vi "log analysis_gps.vi"() -> ()   [LabVIEW 2019] (continued)
0.0929,0.0781,0.0970,0.1019,4.9840,0f000001,0*955fd833\n\t", "INSPVAXA,USB3,0,45.5,FINESTEERING,2107,283346.950,02000000,471d,15824;INS_ALIGNMENT_COMPLETE,INS_RTKFIXED,37.37118779202,126.72299929144,7.7854,22.3000,0.1003,-0.2796,-0.0183,-0.357856906,-0.723006737,278.633509270,0.4452,0.2974,0.5713,0.1136,0.0929,0.0781,0.0970,0.1019,4.9840,0f000001,0*7a9ec2a9\n\t", "INSPVAXA,USB3,0,50.5,FINESTEERING,2107,283347.450,02000000,471d,15824;INS_ALIGNMENT_COMPLETE,INS_RTKFIXED,37.37118807403,126.72299804089,7.7866,22.3000,0.0443,0.0041,-0.0189,-0.283640975,-0.830626211,278.365442964,0.4458,0.2975,0.5714,0.1138,0.0929,0.0781,0.0970,0.1020,4.9856,0f000001,0*be2d3140\n\t", "INSPVAXA,USB3,0,50.5,FINESTEERING,2107,283347.950,02000000,471d,15824;INS_ALIGNMENT_COMPLETE,INS_RTKFIXED,37.37118820355,126.72299809172,7.7880,22.3000,0.0534,-0.0137,-0.0152,-0.361607249,-0.776179806,278.567052976,0.4458,0.2975,0.5714,0.1138,0.0929,0.0781,0.0970,0.1020,4.9856,0f000001,0*5163b365\n\t", "INSPVAXA,USB3,0,46.0,FINESTEERING,2107,283348.450,02008000,471d,15824;INS_ALIGNMENT_COMPLETE,INS_RTKFIXED,37.37118828288,126.72299813022,7.7895,22.3000,0.0516,-0.0114,-0.0144,-0.362235207,-0.776289694,278.558218042,0.4461,0.2975,0.5714,0.1165,0.0930,0.0781,0.0970,0.1020,4.9871,0f000001,0*00d92e93\n\t", "INSPVAXA,USB3,0,46.0,FINESTEERING,2107,283348.950,02008000,471d,15824;INS_ALIGNMENT_COMPLETE,INS_RTKFIXED,37.37118838277,126.72299797344,7.7907,22.3000,0.0830,-0.1936,-0.0090,-0.388787979,-0.629836380,278.403166075,0.4461,0.2975,0.5714,0.1165,0.0930,0.0781,0.0970,0.1020,4.9871,0f000001,0*b6b1c278\n\t", "INSPVAXA,USB3,0,51.0,FINESTEERING,2107,283349.950,02008000,471d,15824;INS_ALIGNMENT_COMPLETE,INS_RTKFIXED,37.37118888254,126.72299463414,7.7948,22.3000,0.0854,-0.2630,-0.0100,-0.254550899,-0.902565471,278.109588384,0.4487,0.2974,0.5715,0.1138,0.0929,0.0781,0.0970,0.1020,4.9866,0f000001,0*b96721fd\n\t", "INSPVAXA,USB3,0,41.5,FINESTEERING,2107,283350.450,02008000,471d,15824;INS_ALIGNMENT_COMPLETE,INS_RTKFIXED,37.37118910944,126.72299305983,7.7973,22.3000,0.0714,-0.2778,-0.0014,-0.407636090,-0.881408174,277.766499487,0.4482,0.2974,0.5716,0.1138,0.0929,0.0781,0.0970,0.1019,4.9868,0f000001,0*7810372a\n\t", "INSPVAXA,USB3,0,41.5,FINESTEERING,2107,283350.950,02008000,471d,15824;INS_ALIGNMENT_COMPLETE,INS_RTKFIXED,37.37118933104,126.72299159852,7.7984,22.3000,0.0589,-0.1073,-0.0277,-0.435946238,-1.120100302,277.342852709,0.4482,0.2974,0.5716,0.1138,0.0929,0.0781,0.0970,0.1019,4.9868,0f000001,0*557f5e08\n\t", "INSPVAXA,USB3,0,48.0,FINESTEERING,2107,283351.450,02008000,471d,15824;INS_ALIGNMENT_COMPLETE,INS_RTKFIXED,37.37118950550,126.72299029919,7.8000,22.3000,0.0990,-0.3064,-0.0104,-0.387241001,-0.965797752,277.134534078,0.4477,0.2974,0.5716,0.1154,0.0930,0.0781,0.0969,0.1019,4.9873,0f000001,0*28a1b0a6\n\t", "INSPVAXA,USB3,0,48.0,FINESTEERING,2107,283351.950,02008000,471d,15824;INS_ALIGNMENT_COMPLETE,INS_RTKFIXED,37.37118970728,126.72298879350,7.8009,22.3000,0.0887,-0.3141,-0.0094,-0.308827403,-0.793055656,276.866791764,0.4477,0.2974,0.5716,0.1154,0.0930,0.0781,0.0969,0.1019,4.9873,0f000001,0*432182b8\n\t", "INSPVAXA,USB3,0,46.5,FINESTEERING,2107,283352.450,02000000,471d,15824;INS_ALIGNMENT_COMPLETE,INS_RTKFIXED,37.37118992961,126.72298725377,7.8025,22.3000,0.0817,-0.2903,-0.0217,-0.165574678,-0.563955548,276.694478613,0.4493,0.2975,0.5717,0.1140,0.0929,0.0781,0.0969,0.1019,4.9857,0f000001,0*b4fa8a95\n\t", "INSPVAXA,USB3,0,46.5,FINESTEERING,2107,283352.950,02000000,471d,15824;INS_ALIGNMENT_COMPLETE,INS_RTKFIXED,37.37119014973,126.72298564431,7.8034,22.3000,0.0887,-0.3034,-0.0088,-0.249749639,-0.735815642,276.497650420,0.4493,0.2975,0.5717,0.1140,0.0929,0.0781,0.0969,0.1019,4.9857,0f000001,0*88cde8fe\n\t", "INSPVAXA,USB3,0,50.0,FINESTEERING,2107,283353.450,02000000,471d,15824;INS_ALIGNMENT_COMPLETE,INS_RTKFIXED,37.37119037224,126.72298404949,7.8038,22.3000,0.0917,-0.2972,-0.0093,-0.357553897,-0.873995960,276.406472875,0.4475,0.2975,0.5716,0.1142,0.0929,0.0781,0.0969,0.1019,4.9865,0f000001,0*353531bb\n\t", "INSPVAXA,USB3,0,50.0,FINESTEERING,2107,283353.950,02000000,471d,15824;INS_ALIGNMENT_COMPLETE,INS_RTKFIXED,37.37119060721,126.72298249352,7.8036,22.3000,0.0817,-0.2975,-0.0112,-0.379231468,-0.836316691,276.368569220,0.4475,0.2975,0.5716,0.1142,0.0929,0.0781,0.0969,0.1019,4.9865,0f000001,0*a3181148\n\t", "INSPVAXA,USB3,0,49.0,FINESTEERING,2107,283354.450,02000000,471d,15824;INS_ALIGNMENT_COMPLETE,INS_RTKFIXED,37.37119085006,126.72298091760,7.8035,22.3000,0.0864,-0.2917,-0.0131,-0.320651128,-0.949485542,276.343611990,0.4461,0.2976,0.5717,0.1143,0.0929,0.0781,0.0969,0.1019,4.9881,0f000001,0*475d9375\n\t", "INSPVAXA,USB3,0,49.0,FINESTEERING,2107,283354.950,02000000,471d,15824;INS_ALIGNMENT_COMPLETE,INS_RTKFIXED,37.37119110500,126.72297932256,7.8027,22.3000,0.0855,-0.2854,-0.0076,-0.293840157,-0.898732844,276.355365665,0.4461,0.2976,0.5717,0.1143,0.0929,0.0781,0.0969,0.1019,4.9881,0f000001,0*d412aada\n\t", "INSPVAXA,USB3,0,51.0,FINESTEERING,2107,283355.450,02000000,471d,15824;INS_ALIGNMENT_COMPLETE,INS_RTKFIXED,37.37119134712,126.72297778450,7.8025,22.3000,0.0859,-0.2925,-0.0070,-0.311679134,-0.669484708,276.428044465,0.4456,0.2977,0.5720,0.1141,0.0929,0.0782,0.0969,0.1019,4.9893,0f000001,0*f22ce517\n\t", "INSPVAXA,USB3,0,51.0,FINESTEERING,2107,283355.950,02000000,471d,15824;INS_ALIGNMENT_COMPLETE,INS_RTKFIXED,37.37119155988,126.72297664236,7.8028,22.3000,0.0638,-0.2658,-0.0150,-0.345823760,-0.347677441,276.253809925,0.4456,0.2977,0.5720,0.1141,0.0929,0.0782,0.0969,0.1019,4.9893,0f000001,0*f6cf90f8\n\t", "INSPVAXA,USB3,0,48.0,FINESTEERING,2107,283356.450,02000000,471d,15824;INS_ALIGNMENT_COMPLETE,INS_RTKFIXED,37.37119183139,126.72297483094,7.8027,22.3000,0.0833,-0.2731,-0.0206,-0.190515377,-0.472405138,276.460349150,0.4456,0.2978,0.5721,0.1141,0.0929,0.0782,0.0969,0.1019,4.9902,0f000001,0*837c9760\n\t", "INSPVAXA,USB3,0,48.0,FINESTEERING,2107,283356.950,02000000,471d,15824;INS_ALIGNMENT_COMPLETE,INS_RTKFIXED,37.37119206486,126.72297337689,7.8027,22.3000,0.0844,-0.3387,-0.0089,-0.224745369,-0.389441077,276.529400158,0.4456,0.2978,0.5721,0.1141,0.0929,0.0782,0.0969,0.1019,4.9902,0f000001,0*8d83a1f7\n\t", "INSPVAXA,USB3,0,50.5,FINESTEERING,2107,283357.950,02000000,471d,15824;INS_ALIGNMENT_COMPLETE,INS_RTKFIXED,37.37119257424,126.72297012404,7.8046,22.3000,0.0855,-0.3001,-0.0197,-0.382775819,-0.574174795,276.720517942,0.4449,0.2976,0.5721,0.1140,0.0929,0.0782,0.0969,0.1019,4.9910,0f000001,0*b9513c1f\n\t", "INSPVAXA,USB3,0,52.0,FINESTEERING,2107,283358.450,02000000,471d,15824;INS_ALIGNMENT_COMPLETE,INS_RTKFIXED,37.37119284307,126.72296856952,7.8054,22.3000,0.0869,-0.3084,-0.0144,-0.231977358,-0.593220103,276.754254189,0.4446,0.2976,0.5721,0.1139,0.0929,0.0782,0.0969,0.1019,4.9917,0f000001,0*6afd1835\n\t", "INSPVAXA,USB3,0,52.0,FINESTEERING,2107,283360.950,02008000,471d,15824;INS_ALIGNMENT_COMPLETE,INS_RTKFIXED,37.37119413375,126.72296080222,7.8105,22.3000,0.0870,-0.3889,-0.0160,0.035751589,-0.478950637,276.922392689,0.4441,0.2974,0.5721,0.1137,0.0929,0.0782,0.0970,0.1020,4.9937,0f000001,0*c5f9a7d1\n\t", "INSPVAXA,USB3,0,51.0,FINESTEERING,2107,283361.950,02008000,471d,15824;INS_ALIGNMENT_COMPLETE,INS_RTKFIXED,37.37119465571,126.72295762324,7.8089,22.3000,0.0624,-0.2772,-0.0071,-0.112500356,-0.370528410,276.848536432,0.4446,0.2976,0.5722,0.1140,0.0929,0.0782,0.0970,0.1020,4.9950,0f000001,0*34f57e0c\n\t", "INSPVAXA,USB3,0,53.0,FINESTEERING,2107,283362.450,02008000,471d,15824;INS_ALIGNMENT_COMPLETE,INS_RTKFIXED,37.37119492880,126.72295600057,7.8073,22.3000,0.0711,-0.2912,-0.0111,0.131468491,-0.238366748,276.764142698,0.4434,0.2974,0.5719,0.1137,0.0929,0.0782,0.0970,0.1020,4.9960,0f000001,0*e2075610\n\t", "INSPVAXA,USB3,0,45.0,FINESTEERING,2107,283364.950,02000000,471d,15824;INS_ALIGNMENT_COMPLETE,INS_RTKFIXED,37.37119619456,126.72294796893,7.8017,22.3000,0.0616,-0.1768,-0.0159,0.378567506,-0.650059405,275.727416770,0.4438,0.2972,0.5717,0.1136,0.0929,0.0781,0.0970,0.1020,4.9990,0f000001,0*15cf5224\n\t", "INSPVAXA,USB3,0,50.0,FINESTEERING,2107,283365.450,02000000,471d,15824;INS_ALIGNMENT_COMPLETE,INS_RTKFIXED,37.37119642630,126.72294649498,7.8002,22.3000,0.0766,-0.2890,-0.0198,0.558482347,-0.615220653,275.473809484,0.4435,0.2971,0.5716,0.1149,0.0929,0.0782,0.0970,0.1020,5.0004,0f000001,0*3ebc86c2\n\t", "INSPVAXA,USB3,0,50.0,FINESTEERING,2107,283365.950,02000000,471d,15824;INS_ALIGNMENT_COMPLETE,INS_RTKFIXED,37.37119665174,126.72294494158,7.7990,22.3000,0.0716,-0.3103,-0.0171,0.492140051,-0.494452644,275.229300180,0.4435,0.2971,0.5716,0.1149,0.0929,0.0782,0.0970,0.1020,5.0004,0f000001,0*39471351\n\t", "INSPVAXA,USB3,0,50.0,FINESTEERING,2107,283366.450,02000000,471d,15824;INS_ALIGNMENT_COMPLETE,INS_RTKFIXED,37.37119686528,126.72294336052,7.7960,22.3000,0.0816,-0.3018,-0.0151,0.434319121,-0.533460520,274.921153499,0.4443,0.2970,0.5716,0.1134,0.0928,0.0781,0.0970,0.1019,5.0004,0f000001,0*50c9815e\n\t", "INSPVAXA,USB3,0,50.0,FINESTEERING,2107,283366.950,02000000,471d,15824;INS_ALIGNMENT_COMPLETE,INS_RTKFIXED,37.37119708745,126.72294176624,7.7921,22.3000,0.0872,-0.3063,-0.0184,0.501847827,-0.459662834,274.603339422,0.4443,0.2970,0.5716,0.1134,0.0928,0.0781,0.0970,0.1019,5.0004,0f000001,0*071e2a71\n\t", "INSPVAXA,USB3,0,51.5,FINESTEERING,2107,283367.450,02000000,471d,15824;INS_ALIGNMENT_COMPLETE,INS_RTKFIXED,37.37119730646,126.72294018823,7.7897,22.3000,0.0762,-0.3201,-0.0092,0.455189651,-0.424726107,274.340978604,0.4433,0.2970,0.5715,0.1134,0.0928,0.0781,0.0969,0.1019,5.0012,0f000001,0*e5f1ee66\n\t", "INSPVAXA,USB3,0,51.5,FINESTEERING,2107,283367.950,02000000,471d,15824;INS_ALIGNMENT_COMPLETE,INS_RTKFIXED,37.37119753251,126.72293860969,7.7876,22.3000,0.0837,-0.3172,-0.0165,0.501901315,-0.449092823,274.123001325,0.4433,0.2970,0.5715,0.1134,0.0928,0.0781,0.0969,0.1019,5.0012,0f000001,0*973b3c7d\n\t", "INSPVAXA,USB3,0,52.0,FINESTEERING,2107,283368.450,02000000,471d,15824;INS_ALIGNMENT_COMPLETE,INS_RTKFIXED,37.37119773991,126.72293703252,7.7857,22.3000,0.0763,-0.3107,-0.0130,0.507599979,-0.527583312,273.978239871,0.4424,0.2970,0.5714,0.1134,0.0929,0.0781,0.0969,0.1019,5.0025,0f000001,0*0977dbed\n\t", "INSPVAXA,USB3,0,52.0,FINESTEERING,2107,283368.950,02000000,471d,15824;INS_ALIGNMENT_COMPLETE,INS_RTKFIXED,37.37119794751,126.72293547014,7.7834,22.3000,0.0774,-0.3055,-0.0096,0.435923288,-0.448613725,273.801043422,0.4424,0.2970,0.5714,0.1134,0.0929,0.0781,0.0969,0.1019,5.0025,0f000001,0*82a00475\n\t", "INSPVAXA,USB3,0,48.5,FINESTEERING,2107,283369.450,02000000,471d,15824;INS_ALIGNMENT_COMPLETE,INS_RTKFIXED,37.37119813318,126.72293389966,7.7815,22.3000,0.0767,-0.3032,-0.0244,0.361736458,-0.446611692,273.637411763,0.4418,0.2971,0.5713,0.1133,0.0928,0.0781,0.0969,0.1019,5.0040,0f000001,0*7557722f\n\t", "INSPVAXA,USB3,0,48.5,FINESTEERING,2107,283369.950,02000000,471d,15824;INS_ALIGNMENT_COMPLETE,INS_RTKFIXED,37.37119830413,126.72293271861,7.7791,22.3000,0.0693,-0.3514,-0.0262,0.354676713,-0.290741223,273.403270579,0.4418,0.2971,0.5713,0.1133,0.0928,0.0781,0.0969,0.1019,5.0040,0f000001,0*dc07d898\n\t", "INSPVAXA,USB3,0,51.0,FINESTEERING,2107,283370.450,02000000,471d,15824;INS_ALIGNMENT_COMPLETE,INS_RTKFIXED,37.37119850662,126.72293105558,7.7771,22.3000,0.0595,-0.2759,-0.0122,0.499717871,-0.539639528,273.303930409,0.4416,0.2971,0.5713,0.1136,0.0928,0.0781,0.0969,0.1019,5.0055,0f000001,0*54bb0a79\n\t", "INSPVAXA,USB3,0,51.0,FINESTEERING,2107,283370.950,02000000,471d,15824;INS_ALIGNMENT_COMPLETE,INS_RTKFIXED,37.37119870016,126.72292944010,7.7758,22.3000,0.0653,-0.2856,-0.0114,0.438696368,-0.681338677,273.167424084,0.4416,0.2971,0.5713,0.1136,0.0928,0.0781,0.0969,0.1019,5.0055,0f000001,0*647e7aec\n\t", "INSPVAXA,USB3,0,49.5,FINESTEERING,2107,283371.450,02000000,471d,15824;INS_ALIGNMENT_COMPLETE,INS_RTKFIXED,37.37119889562,126.72292784230,7.7739,22.3000,0.0592,-0.2777,-0.0188,0.430914391,-0.804071772,273.160470511,0.4407,0.2971,0.5713,0.1133,0.0928,0.0781,0.0970,0.1019,5.0069,0f000001,0*7216170f\n\t", "INSPVAXA,USB3,0,49.5,FINESTEERING,2107,283371.950,02000000,471d,15824;INS_ALIGNMENT_COMPLETE,INS_RTKFIXED,37.37119909971,126.72292622305,7.7712,22.3000,0.0658,-0.2761,-0.0279,0.370330042,-0.824005995,273.116118143,0.4407,0.2971,0.5713,0.1133,0.0928,0.0781,0.0970,0.1019,5.0069,0f000001,0*a32c8b2e\n\t", "INSPVAXA,USB3,0,45.0,FINESTEERING,2107,283372.450,02008000,471d,15824;INS_ALIGNMENT_COMPLETE,INS_RTKFIXED,37.37119927896,126.72292465996,7.7702,22.3000,0.0660,-0.3016,-0.0255,0.364775106,-0.625908727,273.037477195,0.4411,0.2970,0.5714,0.1133,0.0928,0.0782,0.0970,0.1019,5.0085,0f000001,0*0beb0134\n\t", "INSPVAXA,USB3,0,45.0,FINESTEERING,2107,283372.950,02008000,471d,15824;INS_ALIGNMENT_COMPLETE,INS_RTKFIXED,37.37119946128,126.72292307094,7.7690,22.3000,0.0748,-0.2983,-0.0240,0.262839225,-0.610161608,272.980185551,0.4411,0.2970,0.5714,0.1133,0.0928,0.0782,0.0970,0.1019,5.0085,0f000001,0*152c78c5\n\t", "INSPVAXA,USB3,0,43.5,FINESTEERING,2107,283373.950,02008000,471d,15824;INS_ALIGNMENT_COMPLETE,INS_RTKFIXED,37.37119982399,126.72291987146,7.7651,22.3000,0.0739,-0.3179,-0.0233,0.300302749,-0.690108533,272.938320429,0.4412,0.2969,0.5713,0.1133,0.0928,0.0782,0.0970,0.1019,5.0100,0f000001,0*993f6fee\n\t", "INSPVAXA,USB3,0,50.5,FINESTEERING,2107,283374.450,02008000,471d,15824;INS_ALIGNMENT_COMPLETE,INS_RTKFIXED,37.37119999209,126.72291839607,7.7668,22.3000,0.0594,-0.2174,-0.0147,0.364736898,-0.828751718,272.875534675,0.4410,0.2967,0.5712,0.1132,0.0928,0.0781,0.0969,0.1019,5.0114,0f000001,0*e047289e\n\t", "INSPVAXA,USB3,0,44.5,FINESTEERING,2107,283377.450,02000000,471d,15824;INS_ALIGNMENT_COMPLETE,INS_RTKFIXED,37.37120096948,126.72290890698,7.7646,22.3000,0.0650,-0.3099,-0.0265,0.285363327,-1.158258500,272.876132148,0.4400,0.2965,0.5712,0.1130,0.0929,0.0781,0.0969,0.1018,5.0148,0f000001,0*301623f0\n\t", "INSPVAXA,USB3,0,51.5,FINESTEERING,2107,283380.450,02000000,471d,15824;INS_ALIGNMENT_COMPLETE,INS_RTKFIXED,37.37120187255,126.72289967744,7.7619,22.3000,0.0618,-0.2860,-0.0148,0.133286693,-1.082116386,273.127550287,0.4398,0.2963,0.5712,0.1130,0.0928,0.0781,0.0968,0.1018,5.0173,0f000001,0*f1da128c\n\t", "INSPVAXA,USB3,0,47.5,FINESTEERING,2107,283393.500,02000000,471d,15824;INS_ALIGNMENT_COMPLETE,INS_RTKFIXED,37.37120674691,126.72285844800,7.8363,22.3000,0.0562,-0.2735,-0.0060,-0.936766245,0.447139039,273.783760430,0.4461,0.2973,0.5726,0.1135,0.0929,0.0782,0.0967,0.1016,4.9878,0f000001,0*0929eb09\n\t", "INSPVAXA,USB3,0,48.0,FINESTEERING,2107,283397.000,02008000,471d,15824;INS_ALIGNMENT_COMPLETE,INS_RTKFIXED,37.37120756158,126.72284723555,7.8555,22.3000,0.0154,-0.2918,-0.0108,-0.634674297,-0.085063668,267.337636421,0.4417,0.2975,0.5723,0.1133,0.0929,0.0782,0.0967,0.1016,4.9878,0f000001,0*8fe1902c\n\t", "INSPVAXA,USB3,0,46.0,FINESTEERING,2107,283398.500,02000000,471d,15824;INS_ALIGNMENT_COMPLETE,INS_RTKFIXED,37.37120769045,126.72284269521,7.8578,22.3000,0.0082,-0.2767,-0.0005,-0.866355787,-0.085585905,267.490403578,0.4423,0.2980,0.5726,0.1137,0.0929,0.0782,0.0966,0.1016,4.9900,0f000001,0*ee0dcbd5\n\t", "INSPVAXA,USB3,0,46.0,FINESTEERING,2107,283399.000,02000000,471d,15824;INS_ALIGNMENT_COMPLETE,INS_RTKFIXED,37.37120774226,126.72284145946,7.8578,22.3000,0.0199,-0.3107,0.0000,-0.861107937,-0.016080151,267.485200406,0.4423,0.2980,0.5726,0.1137,0.0929,0.0782,0.0966,0.1016,4.9900,0f000001,0*0e2ee5eb\n\t", "INSPVAXA,USB3,0,49.0,FINESTEERING,2107,283400.500,02008000,471d,15824;INS_ALIGNMENT_COMPLETE,INS_RTKFIXED,37.37120790493,126.72283644279,7.8568,22.3000,0.0415,-0.3200,-0.0102,-0.992860449,-0.204263174,269.501464610,0.4444,0.2986,0.5733,0.1141,0.0930,0.0783,0.0966,0.1016,4.9910,0f000001,0*94df5475\n\t", "INSPVAXA,USB3,0,51.0,FINESTEERING,2107,283401.500,02008000,471d,15824;INS_ALIGNMENT_COMPLETE,INS_RTKFIXED,37.37120822785,126.72283327218,7.8567,22.3000,0.0378,-0.2848,0.0013,-0.896017543,0.041472970,274.456577076,0.4448,0.2985,0.5735,0.1139,0.0930,0.0783,0.0966,0.1016,4.9907,0f000001,0*a1fc700f\n\t", "INSPVAXA,USB3,0,51.0,FINESTEERING,2107,283402.000,02008000,471d,15824;INS_ALIGNMENT_COMPLETE,INS_RTKFIXED,37.37120847864,126.72283165681,7.8567,22.3000,0.0753,-0.3061,0.0004,-0.849514538,-0.111394273,277.112069112,0.4448,0.2985,0.5735,0.1139,0.0930,0.0783,0.0966,0.1016,4.9907,0f000001,0*e592cbf0\n\t", "INSPVAXA,USB3,0,40.0,FINESTEERING,2107,283402.500,02008000,471d,15824;INS_ALIGNMENT_COMPLETE,INS_RTKFIXED,37.37120871914,126.72283047198,7.8552,22.3000,0.0392,-0.0732,-0.0063,-0.879415981,-0.139080353,278.991486756,0.4452,0.2985,0.5736,0.1139,0.0932,0.0783,0.0967,0.1016,4.9892,0f000001,0*49d1c048\n\t", "INSPVAXA,USB3,0,40.0,FINESTEERING,2107,283403.000,02008000,471d,15824;INS_ALIGNMENT_COMPLETE,INS_RTKFIXED,37.37120908297,126.72282892192,7.8525,22.3000,0.0902,-0.2460,-0.0094,-0.757562601,-0.250041594,280.800208389,0.4452,0.2985,0.5736,0.1139,0.0932,0.0783,0.0967,0.1016,4.9892,0f000001,0*49bd1315\n\t", "INSPVAXA,USB3,0,49.5,FINESTEERING,2107,283403.500,02008000,471d,15824;INS_ALIGNMENT_COMPLETE,INS_RTKFIXED,37.37120946303,126.72282732667,7.8498,22.3000,0.0944,-0.2806,-0.0193,-0.668842152,-0.504747549,282.253589377,0.4448,0.2984,0.5737,0.1136,0.0933,0.0783,0.0967,0.1016,4.9866,0f000001,0*5936c3a3\n\t", "INSPVAXA,USB3,0,44.5,FINESTEERING,2107,283404.500,02000000,471d,15824;INS_ALIGNMENT_COMPLETE,INS_RTKFIXED,37.37121031708,126.72282412618,7.8426,22.3000,0.0922,-0.2745,-0.0175,-0.508504474,-0.605332941,283.953665433,0.4448,0.2984,0.5737,0.1137,0.0932,0.0783,0.0967,0.1016,4.9838,0f000001,0*f5451d9e\n\t", "INSPVAXA,USB3,0,43.5,FINESTEERING,2107,283405.500,02000000,471d,15824;INS_ALIGNMENT_COMPLETE,INS_RTKFIXED,37.37121122876,126.72282101701,7.8318,22.3000,0.1002,-0.2755,-0.0247,-0.139047561,-0.305791959,284.480251115,0.4442,0.2983,0.5736,0.1136,0.0932,0.0782,0.0967,0.1016,4.9810,0f000001,0*98e81a7f\n\t", "INSPVAXA,USB3,0,43.5,FINESTEERING,2107,283406.000,02000000,471d,15824;INS_ALIGNMENT_COMPLETE,INS_RTKFIXED,37.37121169397,126.72281951047,7.8268,22.3000,0.1108,-0.2868,-0.0208,0.099651120,-0.291418852,284.605342241,0.4442,0.2983,0.5736,0.1136,0.0932,0.0782,0.0967,0.1016,4.9810,0f000001,0*55374de0\n\t", "INSPVAXA,USB3,0,49.5,FINESTEERING,2107,283406.500,02000000,471d,15824;INS_ALIGNMENT_COMPLETE,INS_RTKFIXED,37.37121212971,126.72281808061,7.8238,22.3000,0.1054,-0.2584,-0.0109,0.137601109,-0.336757445,284.673154927,0.4438,0.2982,0.5735,0.1136,0.0935,0.0782,0.0967,0.1016,4.9790,0f000001,0*e60377c5\n\t", "INSPVAXA,USB3,0,49.5,FINESTEERING,2107,283407.000,02000000,471d,15824;INS_ALIGNMENT_COMPLETE,INS_RTKFIXED,37.37121262713,126.72281640166,7.8194,22.3000,0.1069,-0.3011,-0.0264,0.109820957,-0.453228449,284.767303943,0.4438,0.2982,0.5735,0.1136,0.0935,0.0782,0.0967,0.1016,4.9790,0f000001,0*3f427643\n\t", "INSPVAXA,USB3,0,48.0,FINESTEERING,2107,283407.500,02000000,471d,15824;INS_ALIGNMENT_COMPLETE,INS_RTKFIXED,37.37121306195,126.72281499649,7.8146,22.3000,0.1240,-0.3347,-0.0132,0.207501666,-0.436324558,284.580204536,0.4442,0.2982,0.5735,0.1137,0.0934,0.0782,0.0967,0.1017,4.9771,0f000001,0*8c70faff\n\t", "INSPVAXA,USB3,0,48.0,FINESTEERING,2107,283408.000,02000000,471d,15824;INS_ALIGNMENT_COMPLETE,INS_RTKFIXED,37.37121354821,126.72281341269,7.8101,22.3000,0.1116,-0.3074,-0.0226,0.525843943,-0.411708262,284.163389107,0.4442,0.2982,0.5735,0.1137,0.0934,0.0782,0.0967,0.1017,4.9771,0f000001,0*c1d0c0d0\n\t", "INSPVAXA,USB3,0,44.0,FINESTEERING,2107,283408.500,02000000,471d,15824;INS_ALIGNMENT_COMPLETE,INS_RTKFIXED,37.37121398943,126.72281189680,7.8055,22.3000,0.1138,-0.2746,-0.0275,0.675393790,-0.337920064,283.271814178,0.4441,0.2981,0.5734,0.1138,0.0936,0.0782,0.0967,0.1017,4.9759,0f000001,0*ad4dbf0b\n\t", "INSPVAXA,USB3,0,44.0,FINESTEERING,2107,283409.000,02000000,471d,15824;INS_ALIGNMENT_COMPLETE,INS_RTKFIXED,37.37121442754,126.72281035382,7.7998,22.3000,0.1067,-0.2915,-0.0280,0.822552391,-0.280575690,282.018938014,0.4441,0.2981,0.5734,0.1138,0.0936,0.0782,0.0967,0.1017,4.9759,0f000001,0*67fc65b3\n\t", "INSPVAXA,USB3,0,49.0,FINESTEERING,2107,283409.500,02000000,471d,15824;INS_ALIGNMENT_COMPLETE,INS_RTKFIXED,37.37121478666,126.72280882264,7.7967,22.3000,0.1036,-0.2896,-0.0167,0.817605955,-0.233379824,280.341751622,0.4442,0.2981,0.5733,0.1139,0.0934,0.0782,0.0968,0.1017,4.9750,0f000001,0*d948c100\n\t", "INSPVAXA,USB3,0,49.0,FINESTEERING,2107,283410.000,02000000,471d,15824;INS_ALIGNMENT_COMPLETE,INS_RTKFIXED,37.37121511578,126.72280728000,7.7945,22.3000,0.0801,-0.2984,-0.0279,0.678250969,-0.053144715,278.846138365,0.4442,0.2981,0.5733,0.1139,0.0934,0.0782,0.0968,0.1017,4.9750,0f000001,0*ea5c4675\n\t", "INSPVAXA,USB3,0,50.0,FINESTEERING,2107,283410.500,02000000,471d,15824;INS_ALIGNMENT_COMPLETE,INS_RTKFIXED,37.37121543638,126.72280574107,7.7946,22.3000,0.0881,-0.2945,-0.0308,0.799531851,-0.090684476,277.306863329,0.4440,0.2981,0.5734,0.1139,0.0931,0.0782,0.0968,0.1016,4.9749,0f000001,0*8afda85b\n\t", "INSPVAXA,USB3,0,50.0,FINESTEERING,2107,283411.000,02000000,471d,15824;INS_ALIGNMENT_COMPLETE,INS_RTKFIXED,37.37121573081,126.72280419949,7.7932,22.3000,0.0856,-0.2853,-0.0213,0.874963838,0.088876900,275.787048290,0.4440,0.2981,0.5734,0.1139,0.0931,0.0782,0.0968,0.1016,4.9749,0f000001,0*8eff61ca\n\t", "INSPVAXA,USB3,0,47.0,FINESTEERING,2107,283411.500,02000000,471d,15824;INS_ALIGNMENT_COMPLETE,INS_RTKFIXED,37.37121596120,126.72280262366,7.7899,22.3000,0.0704,-0.2845,-0.0255,0.751254674,0.247689552,274.576260626,0.4438,0.2979,0.5732,0.1139,0.0930,0.0782,0.0968,0.1016,4.9755,0f000001,0*e84a82b6\n\t", "INSPVAXA,USB3,0,47.0,FINESTEERING,2107,283412.000,02000000,471d,15824;INS_ALIGNMENT_COMPLETE,INS_RTKFIXED,37.37121617740,126.72280126848,7.7873,22.3000,0.0873,-0.4025,-0.0234,0.616180414,0.315751061,274.011690427,0.4438,0.2979,0.5732,0.1139,0.0930,0.0782,0.0968,0.1016,4.9755,0f000001,0*aa33c281\n\t", "INSPVAXA,USB3,0,49.0,FINESTEERING,2107,283412.500,02000000,471d,15824;INS_ALIGNMENT_COMPLETE,INS_RTKFIXED,37.37121638911,126.72279968745,7.7862,22.3000,0.0846,-0.3281,-0.0274,0.679733503,0.333649216,273.348704844,0.4441,0.2978,0.5733,0.1135,0.0929,0.0782,0.0967,0.1016,4.9761,0f000001,0*b2c3b0d0\n\t", "INSPVAXA,USB3,0,49.0,FINESTEERING,2107,283413.000,02000000,471d,15824;INS_ALIGNMENT_COMPLETE,INS_RTKFIXED,37.37121660586,126.72279809431,7.7843,22.3000,0.0703,-0.2977,-0.0214,0.740409973,0.249491929,272.781944471,0.4441,0.2978,0.5733,0.1135,0.0929,0.0782,0.0967,0.1016,4.9761,0f000001,0*f60b4ece\n\t", "INSPVAXA,USB3,0,52.0,FINESTEERING,2107,283413.500,02000000,471d,15824;INS_ALIGNMENT_COMPLETE,INS_RTKFIXED,37.37121678011,126.72279647899,7.7842,22.3000,0.0611,-0.2896,-0.0156,0.541768048,0.276425000,272.440789392,0.4443,0.2978,0.5734,0.1137,0.0930,0.0783,0.0967,0.1016,4.9772,0f000001,0*dee707a2\n\t", "INSPVAXA,USB3,0,52.0,FINESTEERING,2107,283414.000,02000000,471d,15824;INS_ALIGNMENT_COMPLETE,INS_RTKFIXED,37.37121695844,126.72279487453,7.7833,22.3000,0.0562,-0.2987,-0.0221,0.305746211,0.346254228,272.319331007,0.4443,0.2978,0.5734,0.1137,0.0930,0.0783,0.0967,0.1016,4.9772,0f000001,0*5e10dc17\n\t", "INSPVAXA,USB3,0,50.0,FINESTEERING,2107,283414.500,02000000,471d,15824;INS_ALIGNMENT_COMPLETE,INS_RTKFIXED,37.37121711379,126.72279330042,7.7828,22.3000,0.0616,-0.3002,-0.0329,0.276756604,0.384134091,272.213822291,0.4446,0.2977,0.5735,0.1137,0.0931,0.0783,0.0967,0.1016,4.9781,0f000001,0*58d30e64\n\t", "INSPVAXA,USB3,0,50.0,FINESTEERING,2107,283415.000,02000000,471d,15824;INS_ALIGNMENT_COMPLETE,INS_RTKFIXED,37.37121729157,126.72279172002,7.7811,22.3000,0.0636,-0.2842,-0.0222,0.415011946,0.501817180,272.226800833,0.4446,0.2977,0.5735,0.1137,0.0931,0.0783,0.0967,0.1016,4.9781,0f000001,0*6d269faa\n\t", "INSPVAXA,USB3,0,47.5,FINESTEERING,2107,283415.500,02000000,471d,15824;INS_ALIGNMENT_COMPLETE,INS_RTKFIXED,37.37121745091,126.72279017522,7.7808,22.3000,0.0665,-0.2955,-0.0219,0.380400509,0.552941969,272.302095056,0.4463,0.2979,0.5741,0.1141,0.0931,0.0783,0.0967,0.1016,4.9784,0f000001,0*a1df6ecd\n\t", "INSPVAXA,USB3,0,47.5,FINESTEERING,2107,283416.000,02000000,471d,15824;INS_ALIGNMENT_COMPLETE,INS_RTKFIXED,37.37121761561,126.72278863452,7.7803,22.3000,0.0694,-0.2870,-0.0195,0.176632637,0.631844769,272.368772552,0.4463,0.2979,0.5741,0.1141,0.0931,0.0783,0.0967,0.1016,4.9784,0f000001,0*101cc811\n\t", "INSPVAXA,USB3,0,48.5,FINESTEERING,2107,283416.500,02000000,471d,15824;INS_ALIGNMENT_COMPLETE,INS_RTKFIXED,37.37121775832,126.72278713599,7.7826,22.3000,0.0697,-0.2192,-0.0178,0.097264946,0.637535268,272.514997324,0.4476,0.2980,0.5744,0.1141,0.0933,0.0783,0.0967,0.1016,4.9780,0f000001,0*de8fa7bd\n\t", "INSPVAXA,USB3,0,48.5,FINESTEERING,2107,283417.000,02000000,471d,15824;INS_ALIGNMENT_COMPLETE,INS_RTKFIXED,37.37121791673,126.72278556304,7.7837,22.3000,0.0663,-0.3100,-0.0205,0.059332705,0.713618061,272.644367778,0.4476,0.2980,0.5744,0.1141,0.0933,0.0783,0.0967,0.1016,4.9780,0f000001,0*0eada2f0\n\t", "INSPVAXA,USB3,0,49.5,FINESTEERING,2107,283417.500,02000000,471d,15824;INS_ALIGNMENT_COMPLETE,INS_RTKFIXED,37.37121805927,126.72278401761,7.7854,22.3000,0.0733,-0.3034,-0.0199,-0.089736281,0.682506792,272.907308438,0.4484,0.2980,0.5747,0.1140,0.0932,0.0783,0.0967,0.1016,4.9768,0f000001,0*d6901b99\n\t", "INSPVAXA,USB3,0,49.5,FINESTEERING,2107,283418.000,02000000,471d,15824;INS_ALIGNMENT_COMPLETE,INS_RTKFIXED,37.37121822786,126.72278229435,7.7864,22.3000,0.0757,-0.2957,-0.0211,-0.132925530,0.544261576,273.127275115,0.4484,0.2980,0.5747,0.1140,0.0932,0.0783,0.0967,0.1016,4.9768,0f000001,0*048d27a0\n\t", "INSPVAXA,USB3,0,48.5,FINESTEERING,2107,283418.500,02000000,471d,15824;INS_ALIGNMENT_COMPLETE,INS_RTKFIXED,37.37121838802,126.72278063938,7.7901,22.3000,0.0744,-0.3140,-0.0189,-0.074171217,0.383892357,273.451467378,0.4479,0.2973,0.5742,0.1138,0.0931,0.0783,0.0966,0.1015,4.9755,0f000001,0*a7f0c313\n\t", "INSPVAXA,USB3,0,48.5,FINESTEERING,2107,283419.000,02000000,471d,15824;INS_ALIGNMENT_COMPLETE,INS_RTKFIXED,37.37121856246,126.72277896327,7.7932,22.3000,0.0727,-0.3040,-0.0212,-0.024906260,0.224477115,273.793356519,0.4479,0.2973,0.5742,0.1138,0.0931,0.0783,0.0966,0.1015,4.9755,0f000001,0*a3bde9c9\n\t", "INSPVAXA,USB3,0,48.5,FINESTEERING,2107,283419.500,02000000,471d,15824;INS_ALIGNMENT_COMPLETE,INS_RTKFIXED,37.37121873521,126.72277734418,7.7960,22.3000,0.0758,-0.3154,-0.0078,-0.021214683,0.148956013,274.268869002,0.4473,0.2969,0.5737,0.1137,0.0929,0.0783,0.0966,0.1015,4.9747,0f000001,0*df94383f\n\t", "INSPVAXA,USB3,0,48.5,FINESTEERING,2107,283420.000,02000000,471d,15824;INS_ALIGNMENT_COMPLETE,INS_RTKFIXED,37.37121893456,126.72277571347,7.7975,22.3000,0.0783,-0.3033,-0.0206,0.031637504,0.132212699,274.926400235,0.4473,0.2969,0.5737,0.1137,0.0929,0.0783,0.0966,0.1015,4.9747,0f000001,0*9f2f7546\n\t", "DUALANTENNAHEADINGA,USB3,0,49.5,FINESTEERING,2107,283420.500,02000000,d426,15824;SOL_COMPUTED,L1_FLOAT,-1.000000000,234.407104492,43.477504730,0.0,94.985305786,98.100028992,\"631T\",12,5,5,4,04,00,20,03*0ae8aff3\n\t", "INSPVAXA,USB3,0,49.5,FINESTEERING,2107,283421.000,02000000,471d,15824;INS_ALIGNMENT_COMPLETE,INS_RTKFIXED,37.37121936373,126.72277250548,7.7996,22.3000,0.0650,-0.2575,-0.0195,-0.339414237,-0.334723379,276.547401542,0.4463,0.2965,0.5732,0.1137,0.0928,0.0782,0.0966,0.1015,4.9752,0f000001,0*ec1dc2f2\n\t", "INSPVAXA,USB3,0,51.5,FINESTEERING,2107,283421.500,02000000,471d,15824;INS_ALIGNMENT_COMPLETE,INS_RTKFIXED,37.37121958674,126.72277110428,7.8012,22.3000,0.0748,-0.3049,-0.0167,-0.332988455,-0.342081628,277.184622547,0.4456,0.2963,0.5729,0.1138,0.0929,0.0782,0.0966,0.1015,4.9763,0f000001,0*dbd926c2\n\t", "INSPVAXA,USB3,0,51.5,FINESTEERING,2107,283422.000,02000000,471d,15824;INS_ALIGNMENT_COMPLETE,INS_RTKFIXED,37.37121986544,126.72276955202,7.8030,22.3000,0.0826,-0.2892,-0.0063,-0.059772273,-0.284356871,277.924098643,0.4456,0.2963,0.5729,0.1138,0.0929,0.0782,0.0966,0.1015,4.9763,0f000001,0*9e39ca32\n\t", "INSPVAXA,USB3,0,50.0,FINESTEERING,2107,283422.500,02000000,471d,15824;INS_ALIGNMENT_COMPLETE,INS_RTKFIXED,37.37122013933,126.72276801753,7.8064,22.3000,0.0862,-0.2930,-0.0083,0.046604399,-0.149550594,278.523812878,0.4449,0.2961,0.5725,0.1140,0.0927,0.0782,0.0966,0.1015,4.9774,0f000001,0*ad33b229\n\t", "DUALANTENNAHEADINGA,USB3,0,50.0,FINESTEERING,2107,283423.000,02000000,d426,15824;INSUFFICIENT_OBS,NONE,-1.000000000,0.000000000,0.000000000,0.0,0.000000000,0.000000000,\"631T\",14,4,4,3,04,00,20,03*0f5fdb5e\n\t", "DUALANTENNAHEADINGA,USB3,0,47.0,FINESTEERING,2107,283423.500,02000000,d426,15824;INSUFFICIENT_OBS,NONE,-1.000000000,0.000000000,0.000000000,0.0,0.000000000,0.000000000,\"631T\",14,4,4,3,04,00,20,03*ef3cce1d\n\t", "DUALANTENNAHEADINGA,USB3,0,47.0,FINESTEERING,2107,283424.000,02000000,d426,15824;INSUFFICIENT_OBS,NONE,-1.000000000,0.000000000,0.000000000,0.0,0.000000000,0.000000000,\"631T\",14,4,4,3,04,00,20,03*e256c70a\n\t", "INSPVAXA,USB3,0,47.0,FINESTEERING,2107,283424.500,02000000,471d,15824;INS_ALIGNMENT_COMPLETE,INS_RTKFIXED,37.37122139121,126.72276178934,7.8175,22.3000,0.0963,-0.2911,-0.0267,0.160577040,0.027759936,280.115354795,0.4445,0.2959,0.5718,0.1138,0.0927,0.0782,0.0966,0.1015,4.9793,0f000001,0*3cf8e5a0\n\t", "INSPVAXA,USB3,0,47.0,FINESTEERING,2107,283425.000,02000000,471d,15824;INS_ALIGNMENT_COMPLETE,INS_RTKFIXED,37.37122172446,126.72276025086,7.8192,22.3000,0.1007,-0.2909,-0.0258,0.166214730,-0.121164674,280.254709896,0.4445,0.2959,0.5718,0.1138,0.0927,0.0782,0.0966,0.1015,4.9793,0f000001,0*7313d272\n\t", "INSPVAXA,USB3,0,49.5,FINESTEERING,2107,283425.500,02000000,471d,15824;INS_ALIGNMENT_COMPLETE,INS_RTKFIXED,37.37122203664,126.72275876247,7.8214,22.3000,0.1014,-0.2752,-0.0310,0.225701911,-0.169314911,280.367326711,0.4448,0.2959,0.5717,0.1139,0.0927,0.0782,0.0966,0.1015,4.9800,0f000001,0*47093191\n\t", "INSPVAXA,USB3,0,49.5,FINESTEERING,2107,283426.000,02000000,471d,15824;INS_ALIGNMENT_COMPLETE,INS_RTKFIXED,37.37122236568,126.72275725314,7.8225,22.3000,0.1015,-0.2829,-0.0297,0.362209359,-0.363441278,280.451922060,0.4448,0.2959,0.5717,0.1139,0.0927,0.0782,0.0966,0.1015,4.9800,0f000001,0*8f1e70f0\n\t", "INSPVAXA,USB3,0,46.5,FINESTEERING,2107,283426.500,02000000,471d,15824;INS_ALIGNMENT_COMPLETE,INS_RTKFIXED,37.37122268854,126.72275568297,7.8242,22.3000,0.1049,-0.3026,-0.0329,0.482516704,-0.388354216,280.500192779,0.4446,0.2958,0.5715,0.1139,0.0928,0.0782,0.0966,0.1016,4.9804,0f000001,0*3c38bbfe\n\t", "INSPVAXA,USB3,0,46.5,FINESTEERING,2107,283427.000,02000000,471d,15824;INS_ALIGNMENT_COMPLETE,INS_RTKFIXED,37.37122302372,126.72275405383,7.8254,22.3000,0.1035,-0.2991,-0.0114,0.517295198,-0.533849099,280.546073073,0.4446,0.2958,0.5715,0.1139,0.0928,0.0782,0.0966,0.1016,4.9804,0f000001,0*317727c1\n\t", "DUALANTENNAHEADINGA,USB3,0,47.5,FINESTEERING,2107,283427.500,02000000,d426,15824;SOL_COMPUTED,L1_FLOAT,-1.000000000,232.849288940,45.452278137,0.0,33.969039917,39.167930603,\"631T\",14,5,5,3,04,00,20,03*a09f33ea\n\t", "INSPVAXA,USB3,0,47.5,FINESTEERING,2107,283428.000,02000000,471d,15824;INS_ALIGNMENT_COMPLETE,INS_RTKFIXED,37.37122367818,126.72275085270,7.8261,22.3000,0.0923,-0.2777,-0.0130,0.140840960,-0.867034330,280.536212812,0.4440,0.2956,0.5711,0.1139,0.0927,0.0781,0.0966,0.1016,4.9804,0f000001,0*209210a7\n\t", "INSPVAXA,USB3,0,48.5,FINESTEERING,2107,283428.500,02000000,471d,15824;INS_ALIGNMENT_COMPLETE,INS_RTKFIXED,37.37122400199,126.72274933790,7.8267,22.3000,0.0859,-0.2878,-0.0061,0.135588255,-0.903172735,280.268648781,0.4433,0.2955,0.5708,0.1138,0.0926,0.0781,0.0967,0.1016,4.9799,0f000001,0*057639e6\n\t", "INSPVAXA,USB3,0,48.5,FINESTEERING,2107,283429.000,02000000,471d,15824;INS_ALIGNMENT_COMPLETE,INS_RTKFIXED,37.37122433213,126.72274779084,7.8272,22.3000,0.0909,-0.2670,-0.0074,0.199966599,-0.926566199,279.797605539,0.4433,0.2955,0.5708,0.1138,0.0926,0.0781,0.0967,0.1016,4.9799,0f000001,0*cc69b281\n\t", "DUALANTENNAHEADINGA,USB3,0,47.0,FINESTEERING,2107,283429.500,02000000,d426,15824;SOL_COMPUTED,L1_FLOAT,-1.000000000,232.988739014,45.471614838,0.0,34.093307495,39.104740143,\"631T\",13,5,5,3,04,00,20,03*ea83c899\n\t", "INSPVAXA,USB3,0,47.0,FINESTEERING,2107,283430.000,02000000,471d,15824;INS_ALIGNMENT_COMPLETE,INS_RTKFIXED,37.37122492622,126.72274472809,7.8296,22.3000,0.0738,-0.2911,-0.0264,0.111413714,-0.624845931,278.508262088,0.4425,0.2951,0.5706,0.1137,0.0926,0.0781,0.0967,0.1016,4.9798,0f000001,0*f0033656\n\t", "DUALANTENNAHEADINGA,USB3,0,47.5,FINESTEERING,2107,283430.500,02000000,d426,15824;SOL_COMPUTED,L1_FLOAT,-1.000000000,232.754241943,45.457447052,0.0,33.170593262,38.334568024,\"631T\",11,5,5,3,04,00,20,03*6c1747a2\n\t", "DUALANTENNAHEADINGA,USB3,0,47.5,FINESTEERING,2107,283431.000,02000000,d426,15824;INSUFFICIENT_OBS,NONE,-1.000000000,0.000000000,0.000000000,0.0,0.000000000,0.000000000,\"631T\",11,4,4,3,04,00,20,03*770d0ff4\n\t", "DUALANTENNAHEADINGA,USB3,0,49.5,FINESTEERING,2107,283431.500,02000000,d426,15824;SOL_COMPUTED,L1_FLOAT,-1.000000000,232.641693115,45.342384338,0.0,32.806938171,38.312389374,\"631T\",13,5,5,3,04,00,20,03*517ac67c\n\t", "DUALANTENNAHEADINGA,USB3,0,49.5,FINESTEERING,2107,283432.000,02000000,d426,15824;INSUFFICIENT_OBS,NONE,-1.000000000,0.000000000,0.000000000,0.0,0.000000000,0.000000000,\"631T\",12,4,4,3,04,00,20,03*741ccc0d\n\t", "INSPVAXA,USB3,0,48.0,FINESTEERING,2107,283432.500,02000000,471d,15824;INS_ALIGNMENT_COMPLETE,INS_RTKFIXED,37.37122604855,126.72273724644,7.8341,22.3000,0.0724,-0.2733,-0.0174,0.238872948,0.019909284,274.995506864,0.4422,0.2946,0.5700,0.1135,0.0926,0.0781,0.0966,0.1017,4.9822,0f000001,0*dc53e99c\n\t", "INSPVAXA,USB3,0,48.0,FINESTEERING,2107,283433.000,02000000,471d,15824;INS_ALIGNMENT_COMPLETE,INS_RTKFIXED,37.37122625472,126.72273566540,7.8365,22.3000,0.0706,-0.2887,-0.0199,0.361762560,0.060019418,274.681599898,0.4422,0.2946,0.5700,0.1135,0.0926,0.0781,0.0966,0.1017,4.9822,0f000001,0*5afbe29f\n\t", "DUALANTENNAHEADINGA,USB3,0,49.0,FINESTEERING,2107,283433.500,02000000,d426,15824;SOL_COMPUTED,L1_FLOAT,-1.000000000,232.557586670,45.313392639,0.0,32.878929138,38.560791016,\"631T\",14,5,5,3,04,00,20,03*4c22ef33\n\t", "DUALANTENNAHEADINGA,USB3,0,49.0,FINESTEERING,2107,283434.000,02000000,d426,15824;INSUFFICIENT_OBS,NONE,-1.000000000,0.000000000,0.000000000,0.0,0.000000000,0.000000000,\"631T\",14,4,4,3,04,00,20,03*0b1b3d45\n\t", "INSPVAXA,USB3,0,48.5,FINESTEERING,2107,283434.500,02000000,471d,15824;INS_ALIGNMENT_COMPLETE,INS_RTKFIXED,37.37122687551,126.72273086568,7.8419,22.3000,0.0628,-0.2805,-0.0066,0.210765696,0.014229914,274.274045253,0.4430,0.2944,0.5697,0.1136,0.0924,0.0781,0.0965,0.1017,4.9839,0f000001,0*24038eec\n\t", "INSPVAXA,USB3,0,48.5,FINESTEERING,2107,283435.000,02000000,471d,15824;INS_ALIGNMENT_COMPLETE,INS_RTKFIXED,37.37122709127,126.72272927206,7.8444,22.3000,0.0603,-0.2575,-0.0160,0.234010855,-0.149082924,274.318323900,0.4430,0.2944,0.5697,0.1136,0.0924,0.0781,0.0965,0.1017,4.9839,0f000001,0*fa8bdd9d\n\t", "DUALANTENNAHEADINGA,USB3,0,47.5,FINESTEERING,2107,283435.500,02000000,d426,15824;SOL_COMPUTED,L1_FLOAT,-1.000000000,232.551986694,45.441768646,0.0,33.077499390,38.478469849,\"631T\",15,5,5,3,04,00,20,03*23c7ad13\n\t", "DUALANTENNAHEADINGA,USB3,0,47.5,FINESTEERING,2107,283436.000,02000000,d426,15824;INSUFFICIENT_OBS,NONE,-1.000000000,0.000000000,0.000000000,0.0,0.000000000,0.000000000,\"631T\",13,4,4,3,04,00,20,03*d9c0114b\n\t", "INSPVAXA,USB3,0,49.5,FINESTEERING,2107,283436.500,02000000,471d,15824;INS_ALIGNMENT_COMPLETE,INS_RTKFIXED,37.37122770448,126.72272483106,7.8496,22.3000,0.0698,-0.3222,-0.0225,0.214534417,-0.208140841,274.430810047,0.4422,0.2943,0.5696,0.1135,0.0924,0.0781,0.0965,0.1016,4.9853,0f000001,0*0962ac25\n\t", "DUALANTENNAHEADINGA,USB3,0,49.5,FINESTEERING,2107,283437.000,02000000,d426,15824;INSUFFICIENT_OBS,NONE,-1.000000000,0.000000000,0.000000000,0.0,0.000000000,0.000000000,\"631T\",13,4,4,3,04,00,20,03*a2375da9\n\t", "DUALANTENNAHEADINGA,USB3,0,48.0,FINESTEERING,2107,283437.500,02000000,d426,15824;SOL_COMPUTED,L1_FLOAT,-1.000000000,232.550857544,45.494079590,0.0,33.819896698,39.214233398,\"631T\",14,5,5,3,04,00,20,02*42d48a39\n\t", "INSPVAXA,USB3,0,48.0,FINESTEERING,2107,283438.000,02000000,471d,15824;INS_ALIGNMENT_COMPLETE,INS_RTKFIXED,37.37122838376,126.72272002570,7.8486,22.3000,0.0782,-0.3050,-0.0191,0.083473353,-0.332948382,274.747622714,0.4419,0.2943,0.5694,0.1131,0.0924,0.0781,0.0965,0.1016,4.9857,0f000001,0*6bacac53\n\t", "DUALANTENNAHEADINGA,USB3,0,49.0,FINESTEERING,2107,283438.500,02000000,d426,15824;SOL_COMPUTED,L1_FLOAT,-1.000000000,232.562332153,45.365005493,0.0,33.361850739,38.987976074,\"631T\",11,5,5,3,04,00,20,03*1f4f210e\n\t", "DUALANTENNAHEADINGA,USB3,0,49.0,FINESTEERING,2107,283439.000,02000000,d426,15824;INSUFFICIENT_OBS,NONE,-1.000000000,0.000000000,0.000000000,0.0,0.000000000,0.000000000,\"631T\",12,4,4,3,04,00,20,03*4f2c0de0\n\t", "DUALANTENNAHEADINGA,USB3,0,51.0,FINESTEERING,2107,283439.500,02000000,d426,15824;SOL_COMPUTED,L1_FLOAT,-1.000000000,232.643157959,45.412322998,0.0,33.247821808,38.657192230,\"631T\",11,5,5,3,04,00,20,03*dd544601\n\t", "INSPVAXA,USB3,0,51.0,FINESTEERING,2107,283440.000,02000000,471d,15824;INS_ALIGNMENT_COMPLETE,INS_RTKFIXED,37.37122940222,126.72271360028,7.8520,22.3000,0.0872,-0.2908,-0.0205,-0.014661731,-0.065843852,275.380681368,0.4409,0.2942,0.5694,0.1131,0.0924,0.0781,0.0965,0.1015,4.9875,0f000001,0*9c093e2d\n\t", "INSPVAXA,USB3,0,53.5,FINESTEERING,2107,283440.500,02000000,471d,15824;INS_ALIGNMENT_COMPLETE,INS_RTKFIXED,37.37122969334,126.72271197906,7.8553,22.3000,0.0891,-0.2848,-0.0085,0.255978109,0.004480960,275.509182296,0.4400,0.2941,0.5693,0.1129,0.0924,0.0781,0.0965,0.1015,4.9887,0f000001,0*72ef2c5e\n\t", "DUALANTENNAHEADINGA,USB3,0,53.5,FINESTEERING,2107,283441.000,02000000,d426,15824;INSUFFICIENT_OBS,NONE,-1.000000000,0.000000000,0.000000000,0.0,0.000000000,0.000000000,\"631T\",11,4,4,3,04,00,20,03*7d0e658d\n\t", "INSPVAXA,USB3,0,48.5,FINESTEERING,2107,283441.500,02000000,471d,15824;INS_ALIGNMENT_COMPLETE,INS_RTKFIXED,37.37123027907,126.72270867931,7.8601,22.3000,0.0924,-0.3123,-0.0082,0.186564954,-0.323606469,275.889976490,0.4393,0.2940,0.5692,0.1128,0.0924,0.0781,0.0965,0.1014,4.9899,0f000001,0*5c22d510\n\t", "DUALANTENNAHEADINGA,USB3,0,48.5,FINESTEERING,2107,283442.000,02000000,d426,15824;INSUFFICIENT_OBS,NONE,-1.000000000,0.000000000,0.000000000,0.0,0.000000000,0.000000000,\"631T\",12,4,4,3,04,00,20,03*81e60f26\n\t", "DUALANTENNAHEADINGA,USB3,0,47.0,FINESTEERING,2107,283442.500,02000000,d426,15824;SOL_COMPUTED,L1_FLOAT,-1.000000000,232.738845825,45.537025452,0.0,33.851745605,38.946140289,\"631T\",12,5,5,3,04,00,20,03*fd84ab6f\n\t", "DUALANTENNAHEADINGA,USB3,0,47.0,FINESTEERING,2107,283443.000,02000000,d426,15824;INSUFFICIENT_OBS,NONE,-1.000000000,0.000000000,0.000000000,0.0,0.000000000,0.000000000,\"631T\",12,4,4,3,04,00,20,03*cb2f73ac\n\t", "DUALANTENNAHEADINGA,USB3,0,50.0,FINESTEERING,2107,283443.500,02000000,d426,15824;SOL_COMPUTED,L1_FLOAT,-1.000000000,232.711517334,45.470851898,0.0,33.751167297,39.018550873,\"631T\",12,5,5,3,04,00,20,03*51b2f499\n\t", "DUALANTENNAHEADINGA,USB3,0,50.0,FINESTEERING,2107,283444.000,02000000,d426,15824;INSUFFICIENT_OBS,NONE,-1.000000000,0.000000000,0.000000000,0.0,0.000000000,0.000000000,\"631T\",13,4,4,3,04,00,20,03*f1c4efa0\n\t", "DUALANTENNAHEADINGA,USB3,0,48.0,FINESTEERING,2107,283444.500,02000000,d426,15824;INSUFFICIENT_OBS,NONE,-1.000000000,0.000000000,0.000000000,0.0,0.000000000,0.000000000,\"631T\",13,4,4,3,04,00,20,03*63cc647c\n\t", "DUALANTENNAHEADINGA,USB3,0,48.0,FINESTEERING,2107,283445.000,02000000,d426,15824;INSUFFICIENT_OBS,NONE,-1.000000000,0.000000000,0.000000000,0.0,0.000000000,0.000000000,\"631T\",13,4,4,3,04,00,20,03*d90771fc\n\t", "INSPVAXA,USB3,0,43.5,FINESTEERING,2107,283445.500,02000000,471d,15824;INS_ALIGNMENT_COMPLETE,INS_RTKFIXED,37.37123259759,126.72269590770,7.8782,22.3000,0.0945,-0.3330,-0.0049,0.334033623,-0.428396374,276.205094266,0.4384,0.2941,0.5693,0.1131,0.0924,0.0780,0.0965,0.1014,4.9958,0f000001,0*eef193fc\n\t", "DUALANTENNAHEADINGA,USB3,0,43.5,FINESTEERING,2107,283446.000,02000000,d426,15824;INSUFFICIENT_OBS,NONE,-1.000000000,0.000000000,0.000000000,0.0,0.000000000,0.000000000,\"631T\",12,4,4,3,04,00,20,03*d5fed84d\n\t", "INSPVAXA,USB3,0,50.0,FINESTEERING,2107,283446.500,02000000,471d,15824;INS_ALIGNMENT_COMPLETE,INS_RTKFIXED,37.37123311226,126.72269261048,
